vi "HGF_FGV_Delete.appendData2Variant.vi"(0 "initData":variant, 2 "index":u32, 3 "nofObjects2Delete":u32, 5 "error in (no error)":errorcluster) -> (14 "dup initData":variant, 19 "error out":errorcluster)   [LabVIEW 2012, in "HGF_FGV.lvlib" / "HGF_FGV_Delete.lvclass"]
doc: "Append object initialization data to Variant as attribute."
uses:
  HGF_FGV_Delete.lvclass
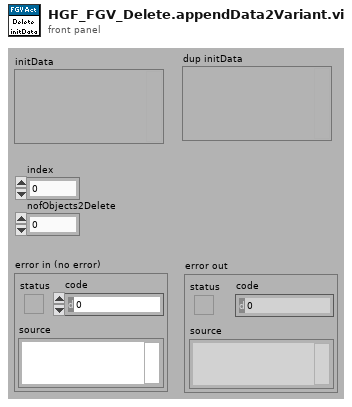
[diagram p1: front panel]
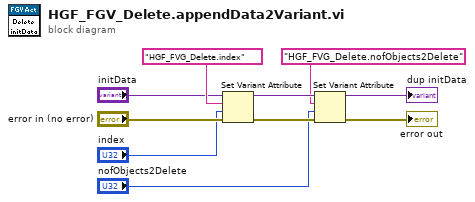
[diagram p0: block diagram]
diagram:
  n1 = Set Variant Attribute(Variant="initData", name="HGF_FVG_Delete.index", value="index", error in="error in (no error)") -> (Variant out=w7:variant, error out=w4:errorcluster)  [unwired: 1 out]
  n2 = Set Variant Attribute(Variant=w7, name="HGF_FVG_Delete.nofObjects2Delete", value="nofObjects2Delete", error in=w4) -> (Variant out=→"dup initData":variant, error out=→"error out":errorcluster)  [unwired: 1 out]
